vi "Test Library Icon Tag.vi"(11 "Test Case In":refnum<class "Library Icon Data.lvclass">) -> (0 "error out":errorcluster, 3 "Test Case Out":refnum<class "Library Icon Data.lvclass">)   [LabVIEW 2020, in "Library Icon Data.lvclass"]
doc: "Saves a library in many different versions (20.0 to current) and verifies the correct tag was used to save the library icon data.\n\nA temporary file is created and deleted as part of this test."
uses:
  Library Icon Data.lvclass
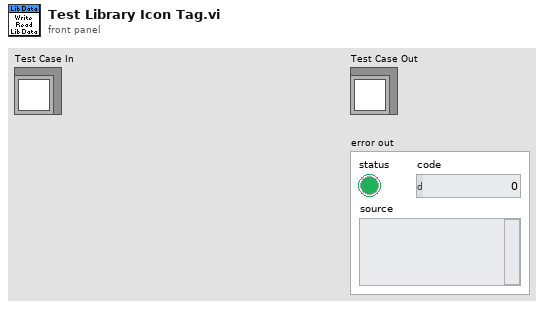
[diagram p1: front panel]
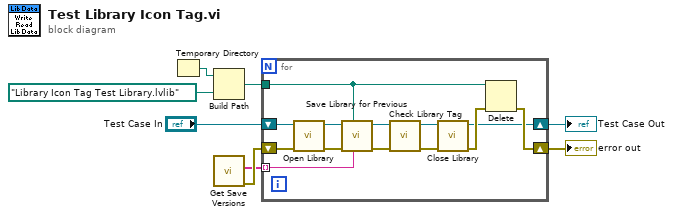
[diagram p0: block diagram]
diagram:
  n1 = Temporary Directory() -> (w6:path)
  n2 = Build Path(base path=w6, name or relative path=path "Library Icon Tag Test Library.lvlib") -> (appended path=w3:path)
  n3 = call "Get Save Versions.vi"() -> ("error out"=w8:errorcluster, "Test Versions"=w4:string[])  [unwired: 10 in]
  n4 = for {
    shift-right: [w18] -> w7
    shift-left: w8 -> [w17]
    shift-right: [w11] -> w2
    shift-left: "Test Case In" -> [w10]
    tunnel: w4 -> [w15] mode=indexing
    tunnel: w3 -> [w12]
    n5 = call "Open Library.vi"("error in"=w17, "Library Icon Data in"=w10) -> ("error out"=w16:errorcluster, "Library Icon Data out"=w9:refnum<class "Library Icon Data.lvclass">)  [unwired: 8 in]
    n6 = call "Save Library for Previous.vi"("Save Version"=w15, "Library Path"=w12, "error in"=w16, "Library Icon Data in"=w9) -> ("error out"=w21:errorcluster, "Library Icon Data out"=w14:refnum<class "Library Icon Data.lvclass">)  [unwired: 6 in]
    n7 = call "Check Library Tag.vi"("error in"=w21, "Library Icon Data in"=w14) -> ("error out"=w19:errorcluster, "Library Icon Data out"=w13:refnum<class "Library Icon Data.lvclass">)  [unwired: 8 in]
    n8 = call "Close Library.vi"("error in"=w19, "Library Icon Data in"=w13) -> ("error out"=w20:errorcluster, "Library Icon Data out"=w11:refnum<class "Library Icon Data.lvclass">)  [unwired: 8 in]
    n9 = Delete(path (use dialog)=w12, error in=w20) -> (error out=w18:errorcluster)  [unwired: 3 in, 2 out]
  }
  "Test Case Out" <- w2
  "error out" <- w7
